vi "Format Log to String.vi"(10 "Log Packet":T1, 11 "HTML File Format in":refnum<class "HTML File Format.lvclass">) -> (2 "Log Entry":string, 3 "HTML File Format out":refnum<class "HTML File Format.lvclass">)   [LabVIEW 2019, in "HTML File Format.lvclass"]
uses:
  <vilib>/gpm_packages/@cs/event-logger/Source/HTML File Sink/HTML File Format.lvclass
  <vilib>/gpm_packages/@cs/event-logger/Source/Composed Log/Types/Log Packet.ctl
  <vilib>/gpm_packages/@cs/event-logger/Source/Composed Log/Types/Log Level.ctl
  <vilib>/gpm_packages/@cs/event-logger/Source/Composed Log/Composed Log.lvlib
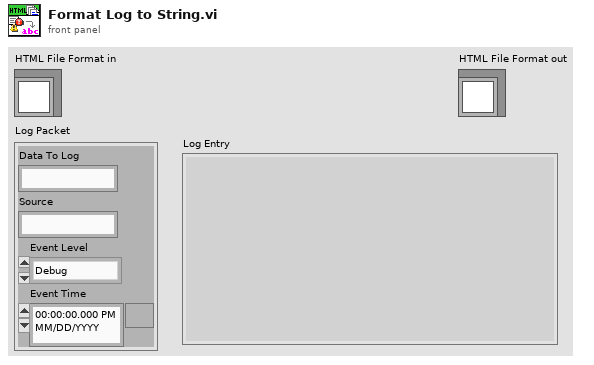
[diagram p1: front panel]
types:
  T1 = typedef "Composed Log.lvlib/Log Packet.ctl" = cluster{"Data To Log":string, "Source":string, "Event Level":T2, "Event Time":timestamp}
  T2 = typedef "Composed Log.lvlib/Log Level.ctl" = enum16{"Debug", "Info", "Warning", "Error", "Critical"}
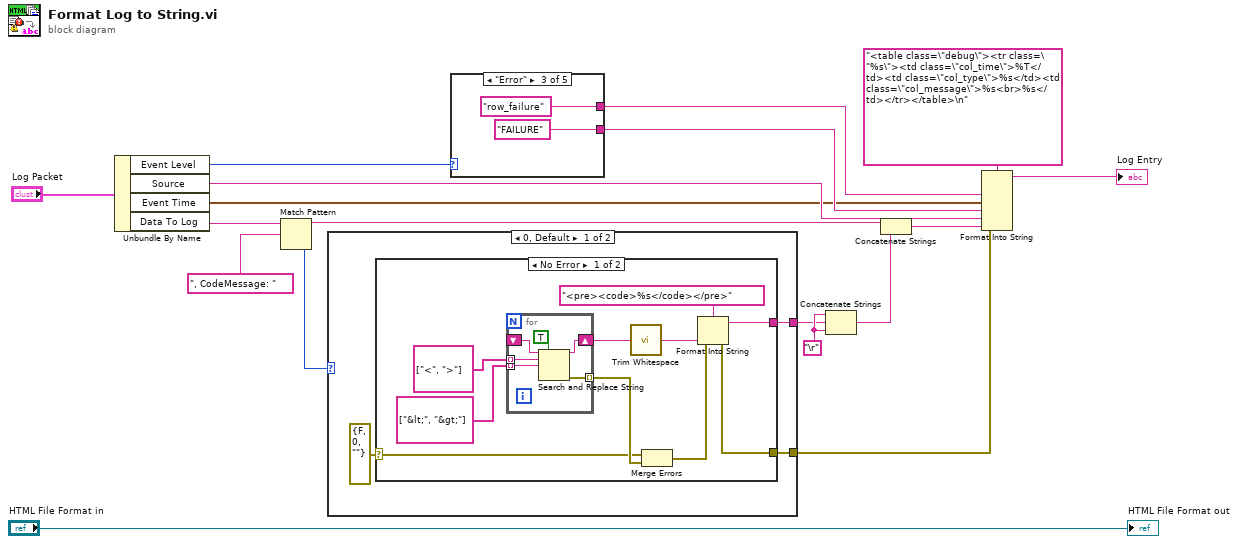
[diagram p0: block diagram]
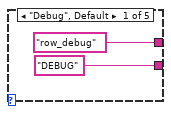
[diagram p4: hidden frame]
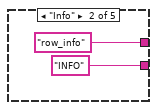
[diagram p5: hidden frame]
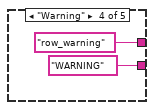
[diagram p6: hidden frame]
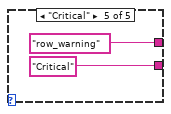
[diagram p7: hidden frame]
diagram:
  w8 = "\r"
  n1 = Unbundle By Name("Log Packet") -> ("Event Level"=w1:T2, "Source"=w15:string, "Event Time"=w4:timestamp, "Data To Log"=w11:string)
  n2 = Match Pattern(string=w11, regular expression=", CodeMessage: ") -> (before substring=w13:string, offset past match=w6:i32)  [unwired: 1 in, 2 out]
  n3 = case shown="0, Default" w6 {
    tunnel: [w21 _] -> w2
    tunnel: [w20 _] -> w7
    frame 0, Default {
      n4 = case shown="No Error" errorcluster {"status"=FALSE, "code"=0, "source"=""} ("error IO") {
        selector: errorcluster {"status"=FALSE, "code"=0, "source"=""} ("error IO") -> [w30 w38]
        tunnel: [w26 w38] -> w21
        tunnel: [w23 _] -> w20
        frame No Error {
          n5 = for {
            tunnel: [w35] -> w31 mode=indexing
            tunnel: string[] ["&lt;", "&gt;"] -> [w34] mode=indexing
            tunnel: string[] ["<", ">"] -> [w33] mode=indexing
            shift-right: [w32] -> w24
            shift-left: _ -> [w36]
            n6 = Search and Replace String(replace all?=TRUE ("replace all? (F)"), input string=w36, search string=w33, replace string=w34) -> (result string=w32:string, error out=w35:errorcluster)  [unwired: 4 in, 2 out]
          }
          n7 = call <vilib>:"Trim Whitespace.vi"("string"=w24) -> ("trimmed string"=w22:string)  [unwired: 1 in]
          n8 = Merge Errors(w30, w31) -> (w27:errorcluster)
          n9 = Format Into String(format string="<pre><code>%s</code></pre>", error in=w27, w22) -> (resulting string=w23:string, error out=w26:errorcluster)  [unwired: 1 in]
        }
        frame Error {
        }
      }
    }
    frame -1 {
    }
  }
  n10 = case shown="\"Error\"" w1 {
    tunnel: ["row_debug" "row_info" "row_failure" "row_warning" "row_warning"] -> w17
    tunnel: ["DEBUG" "INFO" "FAILURE" "WARNING" "Critical"] -> w16
    frame "Debug", Default {
    }
    frame "Info" {
    }
    frame "Error" {
    }
    frame "Warning" {
    }
    frame "Critical" {
    }
  }
  n11 = Concatenate Strings(w8, w7, w8) -> (w5:string)
  n12 = Concatenate Strings(w13, w5) -> (w14:string)
  n13 = Format Into String(format string="<table class=\"debug\"><tr class=\"%s\"><td class=\"col_time\">%T</td><td class=\"col_type\">%s</td><td class=\"col_message\">%s<br>%s</td></tr></table>\n", error in=w2, w17, w4, w16, w15, w14) -> (resulting string=→"Log Entry":string)  [unwired: 1 in, 1 out]
  "HTML File Format out" <- "HTML File Format in"
